vi "Finish.vi"(4 "error in":errorcluster) -> ()   [LabVIEW 2014]
doc: "This VI is called just before exiting. It is expected to close I/O refnum, save collected data, etc."
uses:
  <vilib>/Rock Robotics/WPI/Joystick/WPI_JoystickGetSetRefNum.vi
  <vilib>/Rock Robotics/WPI/Compressor/WPI_CompressorGetSetRefNum.vi
  <vilib>/Rock Robotics/WPI/RobotDrive/WPI_RobotDriveGetSetRefNum.vi
panel:
  # "Finish"
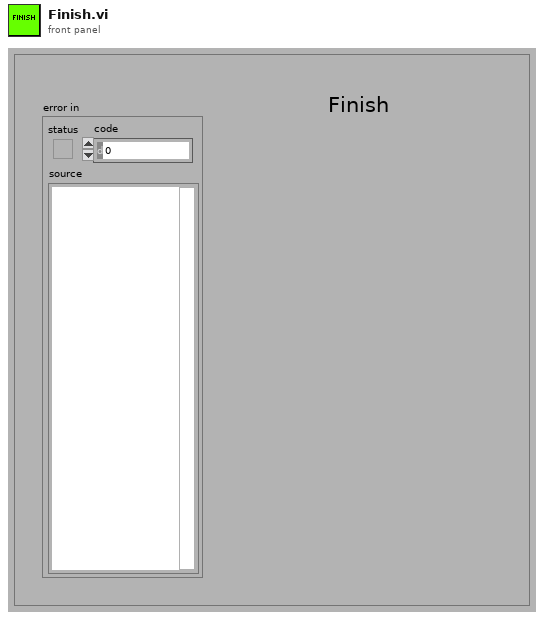
[diagram p1: front panel]
types:
  T1 = typedef "WPI_CompressorDevRef.ctl" = cluster{"DevStatus":errorcluster, "Pneumatics Control Module":u8}
  T2 = typedef "WPI_GyroDevRef.ctl" = cluster{"DevStatus":errorcluster, "Analog Module":T3, "Analog Channel":T4, "Offset":dbl, "Gain (VoltsPerDegree/Second)":dbl}
  T3 = typedef "FPGA_TypedefAnalogModule.ctl" = enum16{"Controller 1"}
  T4 = typedef "FPGA_AIChannel.ctl" = enum8{"AI 0", "AI 1", "AI 2", "AI 3", "AI MXP 0", "AI MXP 1", "AI MXP 2", "AI MXP 3", "Invalid"}
  T5 = typedef "WPI_AnalogChannelDevRef.ctl" = cluster{"DevStatus":errorcluster, "Controller":T3, "Analog Channel":T4}
  T6 = typedef "WPI_SolenoidDevRef.ctl" = cluster{"DevStatus":errorcluster, "Pneumatics Control Module":u8, "Forward Solenoid Channel":T7, "Reverse Solenoid Channel":T7}
  T7 = typedef "WPI_SolenoidChannel.ctl" = enum8{"Solenoid 0", "Solenoid 1", "Solenoid 2", "Solenoid 3", "Solenoid 4", "Solenoid 5", "Solenoid 6", "Solenoid 7", "Invalid"}
  T8 = typedef "WPI_RobotDriveDevRef.ctl" = cluster{"DevStatus":errorcluster, "Motors[]":T9[], "Square Inputs":bool, "Max Output":dbl}
  T9 = typedef "WPI_MotorControlDeviceRef.ctl" = cluster{"DeviceStatus":errorcluster, "Type":T10, "PWM":cluster{"Controller":T11, "PWM Channel":T12, "DeadBand":T13}, "CAN":cluster{"Device Number":u8, "Control Mode":T14, "Semaphore":T15, "Max Vout":dbl, "TalonSRX Control Mode":T16}, "Invert":bool, "TransformRef":T17, "InvTransformRef":T17}
  T10 = typedef "WPI_MotorControlType.ctl" = enum16{"PWM", "CAN", "CANTalonSRX"}
  T11 = typedef "FPGA_TypedefDigitalModule.ctl" = enum16{"Controller 1"}
  T12 = typedef "FPGA_DIOPWMChannel.ctl" = enum8{"PWM 0", "PWM 1", "PWM 2", "PWM 3", "PWM 4", "PWM 5", "PWM 6", "PWM 7", "PWM 8", "PWM 9", "PWM MXP 0", "PWM MXP 1", "PWM MXP 2", "PWM MXP 3", "PWM MXP 4", "PWM MXP 5", "PWM MXP 6", "PWM MXP 7", "PWM MXP 8", "PWM MXP 9", "Invalid"}
  T13 = typedef "WPI_PWMDeadband.ctl" = cluster{"Name":string, "maxPositivePwm":i32, "minPositivePwm":i32, "centerPwm":i32, "maxNegativePwm":i32, "minNegativePwm":i32, "angularRange":u16}
  T14 = typedef "WPI_CANJaguar_ControlMode.ctl" = enum8{"Percent VBus", "Current", "Speed", "Position", "Voltage"}
  T15 = typedef "Semaphore RefNum" = refnum<k1>
  T16 = typedef "WPI_CANTalonSRX_APIControlMode.ctl" = enum8{"Percent VBus", "Speed", "Position", "Slave", "Unchanged / Invalid"}
  T17 = typedef "WPI_PWMTransform_ConPane.ctl" = refnum<vi>
  T18 = typedef "WPI_EncoderDevRef.ctl" = cluster{"DevStatus":errorcluster, "EncoderIndex":T19, "CounterIndex":T20, "DistancePerCount":dbl, "Decoding Type":T21}
  T19 = typedef "FPGA_EncoderIdx.ctl" = enum8{"Enc 0", "Enc 1", "Enc 2", "Enc 3", "Enc 4", "Enc 5", "Enc 6", "Enc 7", "Invalid"}
  T20 = typedef "FPGA_CounterCtrSystemIndex.ctl" = enum8{"Ctr 0", "Ctr 1", "Ctr 2", "Ctr 3", "Ctr 4", "Ctr 5", "Ctr 6", "Ctr 7", "Invalid"}
  T21 = typedef "WPI_EncoderType.ctl" = enum16{"1x", "2x", "4x"}
  T22 = typedef "WPI_JoystickDevRef.ctl" = cluster{"Device":T23}
  T23 = typedef "WPI_JoystickDeviceEnum.ctl" = enum16{"USB 0", "USB 1", "USB 2", "USB 3", "USB 4", "USB 5"}
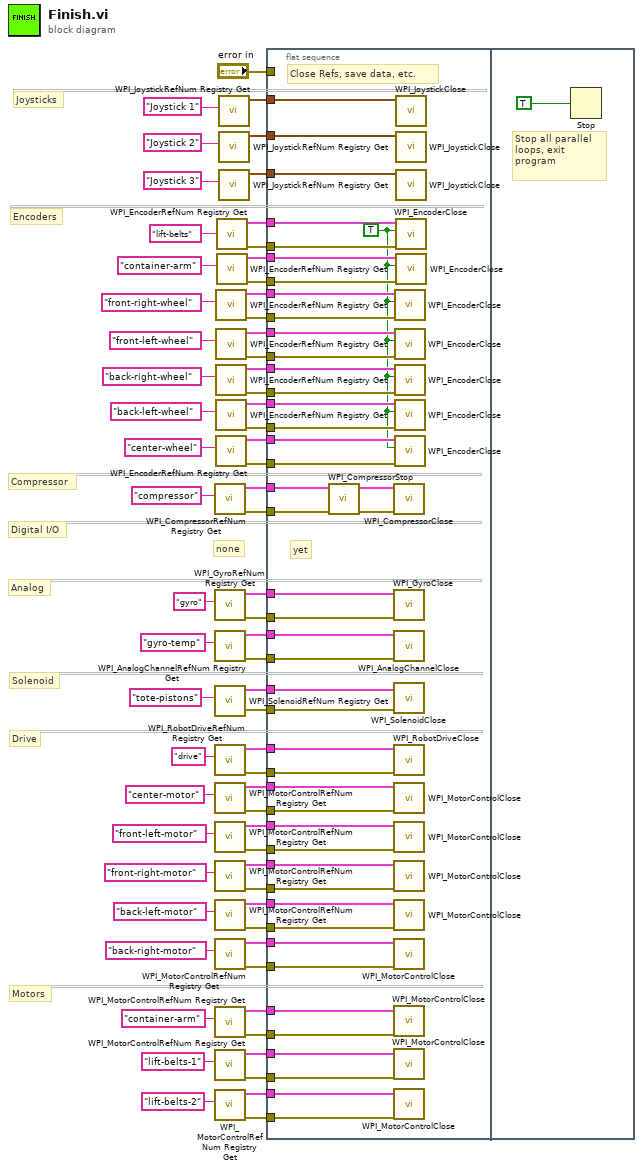
[diagram p0: block diagram]
diagram:
  # "none"
  # "Analog"
  # "Motors"
  # "Drive"
  # "Solenoid"
  # "Digital I/O"
  # "Compressor"
  # "Encoders"
  # "Joysticks"
  n1 = call <vilib>:"WPI_CompressorRefNum Registry Get.vi"("refnum name"="compressor") -> ("error out"=w36:errorcluster, "CompressorDevRef"=w46:T1)  [unwired: 9 in]
  n2 = call <vilib>:"WPI_GyroRefNum Registry Get.vi"("refnum name"="gyro") -> ("error out"=w16:errorcluster, "GyroDevRef"=w17:T2)  [unwired: 9 in]
  n3 = call <vilib>:"WPI_AnalogChannelRefNum Registry Get.vi"("refnum name"="gyro-temp") -> ("error out"=w2:errorcluster, "AIDeviceRef"=w3:T5)  [unwired: 9 in]
  n4 = call <vilib>:"WPI_SolenoidRefNum Registry Get.vi"("refnum name"="tote-pistons") -> ("error out"=w35:errorcluster, "SolenoidDevRef"=w44:T6)  [unwired: 9 in]
  n5 = call <vilib>:"WPI_RobotDriveRefNum Registry Get.vi"("refnum name"="drive") -> ("error out"=w32:errorcluster, "RobotDriveDevRef"=w33:T8)  [unwired: 9 in]
  n6 = call <vilib>:"WPI_MotorControlRefNum Registry Get.vi"("refnum name"="center-motor") -> ("error out"=w29:errorcluster, "MotorControlDevRef"=w30:T9)  [unwired: 9 in]
  n7 = call <vilib>:"WPI_MotorControlRefNum Registry Get.vi"("refnum name"="front-left-motor") -> ("error out"=w15:errorcluster, "MotorControlDevRef"=w14:T9)  [unwired: 9 in]
  n8 = call <vilib>:"WPI_MotorControlRefNum Registry Get.vi"("refnum name"="front-right-motor") -> ("error out"=w9:errorcluster, "MotorControlDevRef"=w8:T9)  [unwired: 9 in]
  n9 = call <vilib>:"WPI_MotorControlRefNum Registry Get.vi"("refnum name"="back-left-motor") -> ("error out"=w10:errorcluster, "MotorControlDevRef"=w11:T9)  [unwired: 9 in]
  n10 = call <vilib>:"WPI_MotorControlRefNum Registry Get.vi"("refnum name"="back-right-motor") -> ("error out"=w6:errorcluster, "MotorControlDevRef"=w5:T9)  [unwired: 9 in]
  n11 = call <vilib>:"WPI_MotorControlRefNum Registry Get.vi"("refnum name"="container-arm") -> ("error out"=w28:errorcluster, "MotorControlDevRef"=w27:T9)  [unwired: 9 in]
  n12 = call <vilib>:"WPI_MotorControlRefNum Registry Get.vi"("refnum name"="lift-belts-1") -> ("error out"=w25:errorcluster, "MotorControlDevRef"=w24:T9)  [unwired: 9 in]
  n13 = call <vilib>:"WPI_MotorControlRefNum Registry Get.vi"("refnum name"="lift-belts-2") -> ("error out"=w20:errorcluster, "MotorControlDevRef"=w21:T9)  [unwired: 9 in]
  n14 = call <vilib>:"WPI_EncoderRefNum Registry Get.vi"("refnum name"="front-right-wheel") -> ("error out"=w41:errorcluster, "EncoderDevRef"=w51:T18)  [unwired: 9 in]
  n15 = call <vilib>:"WPI_EncoderRefNum Registry Get.vi"("refnum name"="front-left-wheel") -> ("error out"=w40:errorcluster, "EncoderDevRef"=w50:T18)  [unwired: 9 in]
  n16 = call <vilib>:"WPI_EncoderRefNum Registry Get.vi"("refnum name"="back-right-wheel") -> ("error out"=w39:errorcluster, "EncoderDevRef"=w49:T18)  [unwired: 9 in]
  n17 = call <vilib>:"WPI_EncoderRefNum Registry Get.vi"("refnum name"="back-left-wheel") -> ("error out"=w38:errorcluster, "EncoderDevRef"=w48:T18)  [unwired: 9 in]
  n18 = call <vilib>:"WPI_EncoderRefNum Registry Get.vi"("refnum name"="center-wheel") -> ("error out"=w37:errorcluster, "EncoderDevRef"=w47:T18)  [unwired: 9 in]
  n19 = call <vilib>:"WPI_EncoderRefNum Registry Get.vi"("refnum name"="lift-belts") -> ("error out"=w43:errorcluster, "EncoderDevRef"=w53:T18)  [unwired: 9 in]
  n20 = call <vilib>:"WPI_EncoderRefNum Registry Get.vi"("refnum name"="container-arm") -> ("error out"=w42:errorcluster, "EncoderDevRef"=w52:T18)  [unwired: 9 in]
  n21 = call <vilib>:"WPI_JoystickRefNum Registry Get.vi"("refnum name"="Joystick 1") -> ("JoystickDevRef"=w66:T22)  [unwired: 1 in, 9 out]
  n22 = call <vilib>:"WPI_JoystickRefNum Registry Get.vi"("refnum name"="Joystick 2") -> ("JoystickDevRef"=w65:T22)  [unwired: 1 in, 9 out]
  n23 = call <vilib>:"WPI_JoystickRefNum Registry Get.vi"("refnum name"="Joystick 3") -> ("JoystickDevRef"=w62:T22)  [unwired: 1 in, 9 out]
  n24 = flat-sequence {
    tunnel: w66 -> [w113]
    tunnel: w65 -> [w112]
    tunnel: w62 -> [w111]
    tunnel: "error in" -> [_]
    tunnel: w53 -> [w110]
    tunnel: w52 -> [w109]
    tunnel: w51 -> [w108]
    tunnel: w50 -> [w107]
    tunnel: w49 -> [w106]
    tunnel: w48 -> [w105]
    tunnel: w47 -> [w101]
    tunnel: w46 -> [w103]
    tunnel: w44 -> [w102]
    tunnel: w43 -> [w100]
    tunnel: w42 -> [w91]
    tunnel: w41 -> [w99]
    tunnel: w40 -> [w98]
    tunnel: w39 -> [w97]
    tunnel: w38 -> [w96]
    tunnel: w37 -> [w95]
    tunnel: w36 -> [w93]
    tunnel: w35 -> [w94]
    tunnel: w33 -> [w88]
    tunnel: w32 -> [w87]
    tunnel: w30 -> [w90]
    tunnel: w29 -> [w89]
    tunnel: w27 -> [w85]
    tunnel: w28 -> [w86]
    tunnel: w24 -> [w83]
    tunnel: w25 -> [w84]
    tunnel: w21 -> [w82]
    tunnel: w20 -> [w81]
    tunnel: w17 -> [w79]
    tunnel: w16 -> [w78]
    tunnel: w14 -> [w76]
    tunnel: w15 -> [w77]
    tunnel: w8 -> [w72]
    tunnel: w9 -> [w73]
    tunnel: w11 -> [w75]
    tunnel: w10 -> [w74]
    tunnel: w5 -> [w70]
    tunnel: w6 -> [w71]
    tunnel: w3 -> [w69]
    tunnel: w2 -> [w68]
    frame #0 {
      w80 = TRUE ("Close Dependencies")
      # "yet"
      # "Close Refs, save data, etc."
      n25 = call <vilib>:"WPI_CompressorStop.vi"("error in (no error)"=w93, "CompressorDevRef"=w103) -> ("error out"=w92:errorcluster, "CompressorDevRef"=w104:T1)  [unwired: 8 in]
      n26 = call <vilib>:"WPI_CompressorClose.vi"("error in (no error)"=w92, "CompressorDevRef"=w104) -> ()  [unwired: 9 in, 1 out]
      n27 = call <vilib>:"WPI_GyroClose.vi"("error in (no error)"=w78, "GyroDevRef"=w79) -> ()  [unwired: 9 in, 1 out]
      n28 = call <vilib>:"WPI_AnalogChannelClose.vi"("error in (no error)"=w68, "AIDeviceRef"=w69) -> ()  [unwired: 9 in, 1 out]
      n29 = call <vilib>:"WPI_SolenoidClose.vi"("error in (no error)"=w94, "SolenoidDevRef"=w102) -> ()  [unwired: 9 in, 1 out]
      n30 = call <vilib>:"WPI_RobotDriveClose.vi"("error in (no error)"=w87, "RobotDriveDevRef"=w88) -> ()  [unwired: 9 in, 1 out]
      n31 = call <vilib>:"WPI_MotorControlClose.vi"("error in (no error)"=w89, "MotorControlDevRef"=w90) -> ()  [unwired: 9 in, 1 out]
      n32 = call <vilib>:"WPI_MotorControlClose.vi"("error in (no error)"=w77, "MotorControlDevRef"=w76) -> ()  [unwired: 9 in, 1 out]
      n33 = call <vilib>:"WPI_MotorControlClose.vi"("error in (no error)"=w73, "MotorControlDevRef"=w72) -> ()  [unwired: 9 in, 1 out]
      n34 = call <vilib>:"WPI_MotorControlClose.vi"("error in (no error)"=w74, "MotorControlDevRef"=w75) -> ()  [unwired: 9 in, 1 out]
      n35 = call <vilib>:"WPI_MotorControlClose.vi"("error in (no error)"=w71, "MotorControlDevRef"=w70) -> ()  [unwired: 9 in, 1 out]
      n36 = call <vilib>:"WPI_MotorControlClose.vi"("error in (no error)"=w86, "MotorControlDevRef"=w85) -> ()  [unwired: 9 in, 1 out]
      n37 = call <vilib>:"WPI_MotorControlClose.vi"("error in (no error)"=w84, "MotorControlDevRef"=w83) -> ()  [unwired: 9 in, 1 out]
      n38 = call <vilib>:"WPI_MotorControlClose.vi"("error in (no error)"=w81, "MotorControlDevRef"=w82) -> ()  [unwired: 9 in, 1 out]
      n39 = call <vilib>:"WPI_EncoderClose.vi"("error in (no error)"=w99, "Close Dependencies"=w80, "EncoderDevRef"=w108) -> ()  [unwired: 8 in, 1 out]
      n40 = call <vilib>:"WPI_EncoderClose.vi"("error in (no error)"=w98, "Close Dependencies"=w80, "EncoderDevRef"=w107) -> ()  [unwired: 8 in, 1 out]
      n41 = call <vilib>:"WPI_EncoderClose.vi"("error in (no error)"=w97, "Close Dependencies"=w80, "EncoderDevRef"=w106) -> ()  [unwired: 8 in, 1 out]
      n42 = call <vilib>:"WPI_EncoderClose.vi"("error in (no error)"=w96, "Close Dependencies"=w80, "EncoderDevRef"=w105) -> ()  [unwired: 8 in, 1 out]
      n43 = call <vilib>:"WPI_EncoderClose.vi"("error in (no error)"=w95, "Close Dependencies"=w80, "EncoderDevRef"=w101) -> ()  [unwired: 8 in, 1 out]
      n44 = call <vilib>:"WPI_JoystickClose.vi"("JoystickDevRef"=w113) -> ()  [unwired: 11 out]
      n45 = call <vilib>:"WPI_JoystickClose.vi"("JoystickDevRef"=w112) -> ()  [unwired: 11 out]
      n46 = call <vilib>:"WPI_JoystickClose.vi"("JoystickDevRef"=w111) -> ()  [unwired: 11 out]
      n47 = call <vilib>:"WPI_EncoderClose.vi"("error in (no error)"=w100, "Close Dependencies"=w80, "EncoderDevRef"=w110) -> ()  [unwired: 8 in, 1 out]
      n48 = call <vilib>:"WPI_EncoderClose.vi"("error in (no error)"=w91, "Close Dependencies"=w80, "EncoderDevRef"=w109) -> ()  [unwired: 8 in, 1 out]
    }
    frame #1 {
      # "Stop all parallel\nloops, exit program"
      n49 = Stop(stop? (T)=TRUE ("Quit")) -> ()
    }
  }
